vi "18_DC Motor_PID_test_3.vi"() -> ()   [LabVIEW 2018]
uses:
  <userlib>/KNR OS 4.0 LabVIEW Toolkit/Type Definition/DC Motor Port.ctl
  <userlib>/KNR OS 4.0 LabVIEW Toolkit/Type Definition/Resource.ctl
panel:
  in  "R Reverse":bool
  in  "Enable Motor 2":bool
  in  "Enable sync":bool=TRUE
  in  "Kp 3":dbl(slide)=0.2 scale=0.0..0.8
  in  "Ki 3":dbl(slide)=0.05 scale=0.0..0.1
  in  "Kd 3":dbl(slide)=0.02 scale=0.0..0.2
  in  "PID sync":bool=TRUE
  out "Speed (+-100%) 2":dbl
  out "Velocity (cm/sec) 2":dbl
  in  "Port 2":T1=5 items=["DS1"=4, "DS2"=5, "DS3"=6, "DS4"=7]
  out "Velocity (cm/sec) Chart 2":dbl(graph)
  out "Desire Velosity (cm/sec) 2":dbl
  in  "Desire Velosity (cm/sec)":dbl=15.0 format="%#_13g"
  in  "F/B switch":bool=TRUE
  in  "Port":T1=4 items=["DS1"=4, "DS2"=5, "DS3"=6, "DS4"=7]
  out "Velocity (cm/sec) Chart":dbl(graph)
  out "Speed (+-100%)":dbl
  in  "Kd":dbl(slide)=0.02 scale=0.0..0.2
  in  "Ki":dbl(slide)=0.05 scale=0.0..0.1
  in  "Kp":dbl(slide)=0.2 scale=0.0..0.8
  in  "stop":bool
  in  "Enable Motor 1":bool
  out "Velocity (cm/sec)":dbl
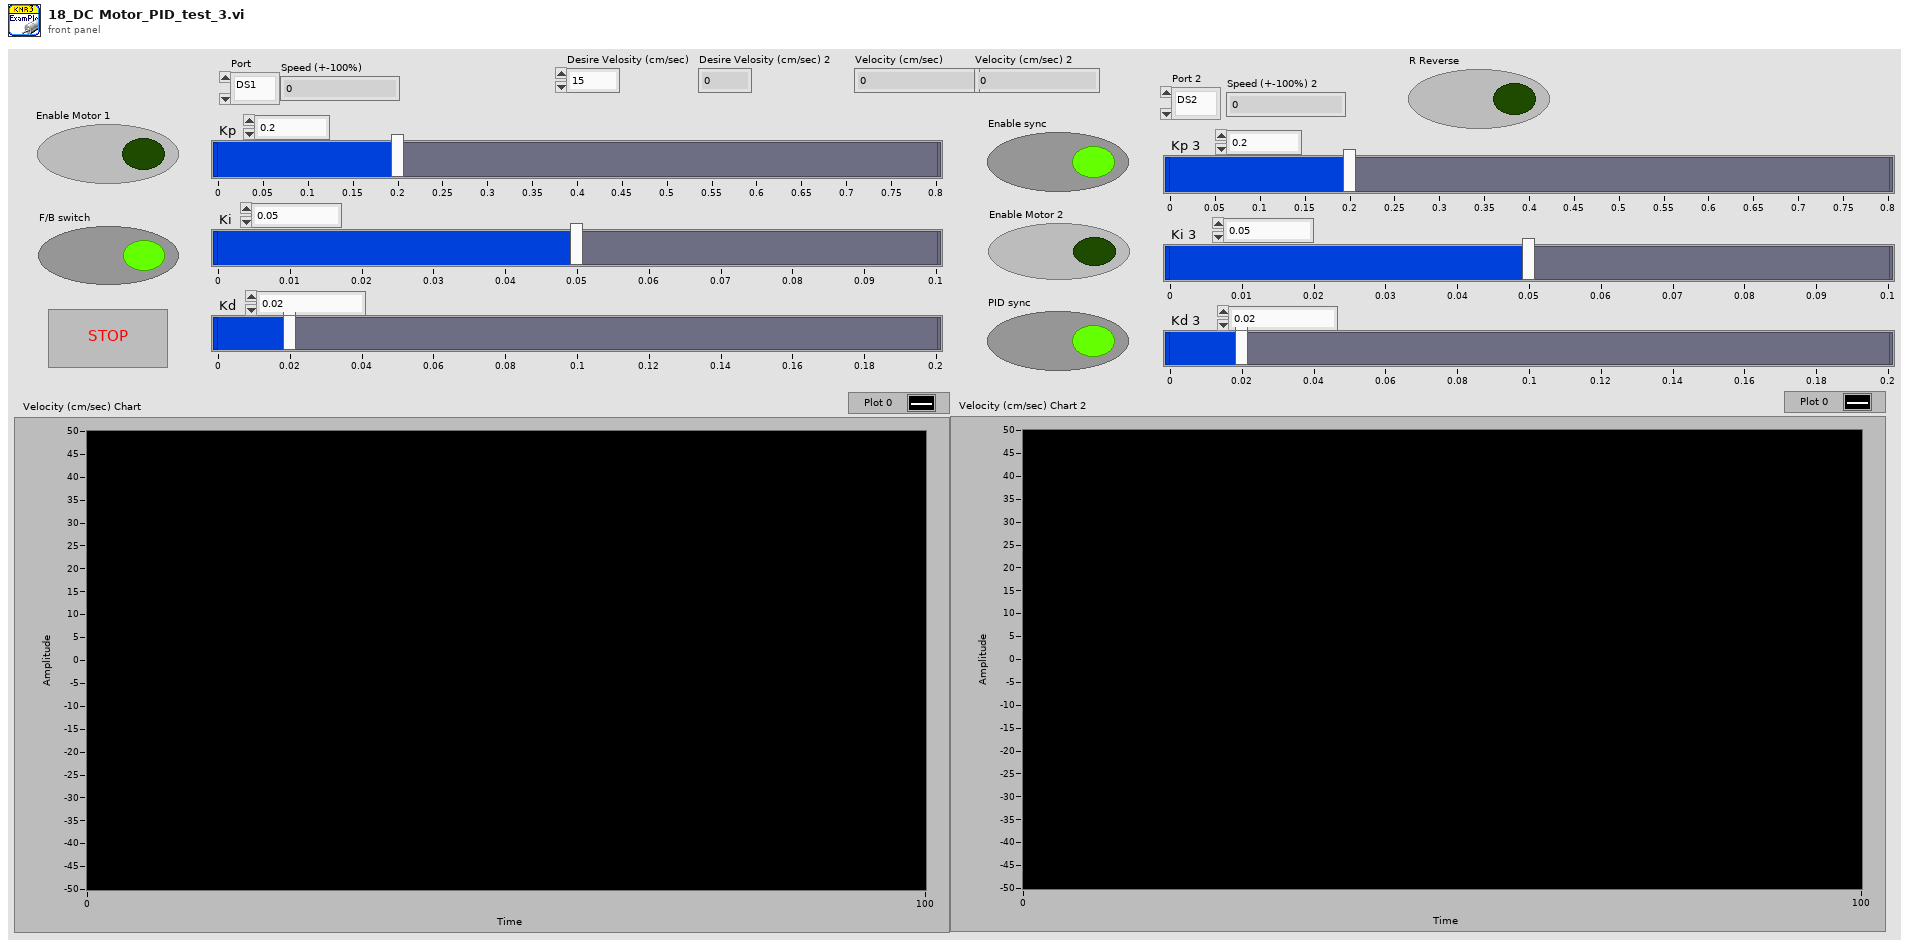
[diagram p1: front panel]
types:
  T1 = typedef "DC Motor Port.ctl" = u16
  T2 = typedef "Resource.ctl" = enum16{"KNRm_DDRC", "KNRm_DDDD", "KNRm_DDDR", "KNRm_DDDC", "KNR", "KNRm_neww"}
  T3 = typedef "KNR3 Reference.ctl" = cluster{"FPGA Session":refnum<class "FPGA Interface Base.lvclass">, "Resource":T2}
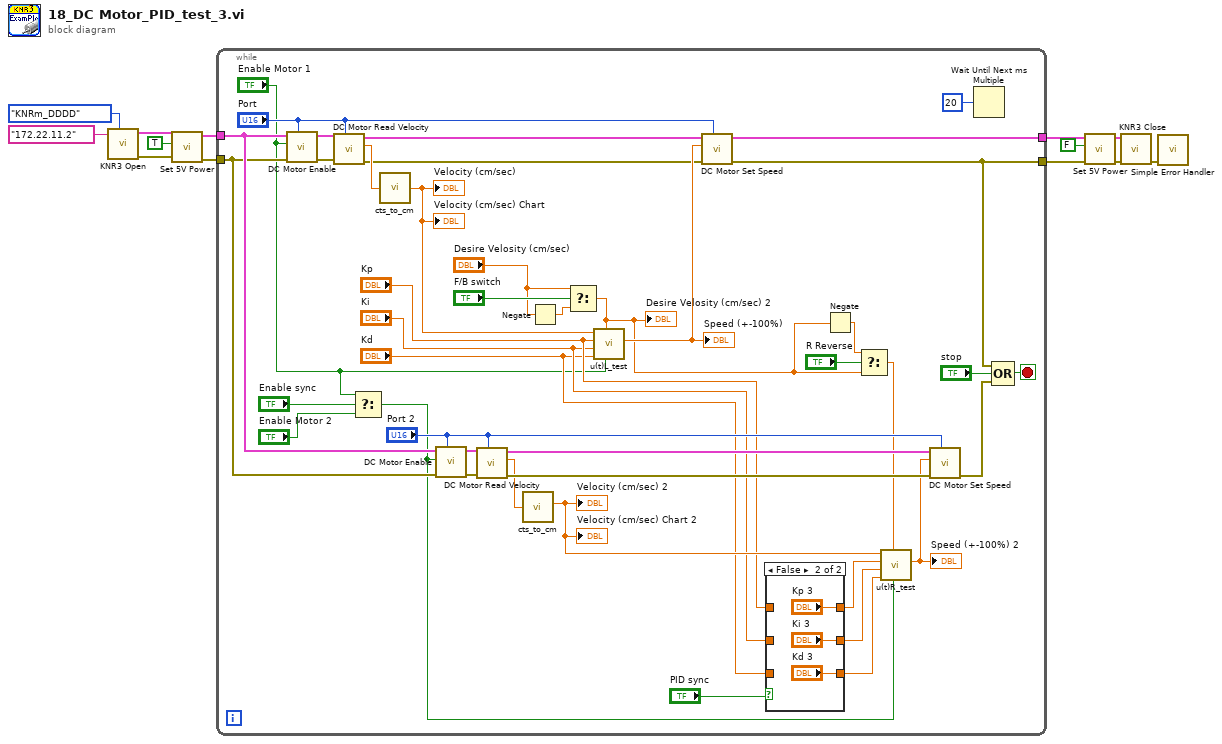
[diagram p0: block diagram]
diagram:
  n1 = call <userlib>:"KNR3 Open.vi"("Resource"=Resource."KNRm_DDDD", "IP"="172.22.11.2") -> ("error out"=w6:errorcluster, "KNR out"=w8:T3)  [unwired: 8 in]
  n2 = call <userlib>:"Set 5V Power.vi"("error in (no error)"=w6, "5V Power(T)"=TRUE ("5V Power"), "KNR in"=w8) -> ("error out"=w10:errorcluster, "KNR out"=w11:T3)  [unwired: 7 in]
  n3 = while {
    tunnel: w11 -> [w36]
    tunnel: w10 -> [w35]
    tunnel: [w47] -> w4
    tunnel: [w46] -> w3
    stop <- w53 stop-if-true
    n4 = call <userlib>:"DC Motor Enable.vi"("Port (DS1)"="Port", "error in (no error)"=w35, "Enable Motor(F)"="Enable Motor 1", "KNR in"=w36) -> ("error out"=w50:errorcluster, "KNR out"=w51:T3)  [unwired: 6 in]
    n5 = call <userlib>:"DC Motor Read Velocity.vi"("Port (DS1)"="Port", "error in (no error)"=w50, "KNR in"=w51) -> ("error out"=w43:errorcluster, "Velocity (cts/sec)"=w49:dbl, "KNR out"=w44:T3)  [unwired: 6 in]
    n6 = Select(t="Enable Motor 1", s="Enable sync", f="Enable Motor 2") -> (s? t:f=w21:bool)
    n7 = call "cts_to_cm.vi"("cts"=w49) -> ("cm"=w28:dbl)
    "Velocity (cm/sec)" <- w28
    "Velocity (cm/sec) Chart" <- w28
    n8 = call <userlib>:"DC Motor Enable.vi"("Port (DS1)"="Port 2", "error in (no error)"=w35, "Enable Motor(F)"=w21, "KNR in"=w36) -> ("error out"=w38:errorcluster, "KNR out"=w37:T3)  [unwired: 6 in]
    n9 = call <userlib>:"DC Motor Read Velocity.vi"("Port (DS1)"="Port 2", "error in (no error)"=w38, "KNR in"=w37) -> ("error out"=w42:errorcluster, "Velocity (cts/sec)"=w39:dbl, "KNR out"=w41:T3)  [unwired: 6 in]
    n10 = call "cts_to_cm.vi"("cts"=w39) -> ("cm"=w31:dbl)
    "Velocity (cm/sec) 2" <- w31
    "Velocity (cm/sec) Chart 2" <- w31
    n11 = Negate(x="Desire Velosity (cm/sec)") -> (-x=w18:dbl)
    n12 = Select(t="Desire Velosity (cm/sec)", s="F/B switch", f=w18) -> (s? t:f=w13:dbl)
    "Desire Velosity (cm/sec) 2" <- w13
    n13 = call "u(t)L_test.vi"("enable"="Enable Motor 1", "Desire Velosity"=w13, "Kd"="Kd", "Ki"="Ki", "Kp"="Kp", "Velocity"=w28) -> ("u(t)"=w45:dbl)  [unwired: 5 in]
    "Speed (+-100%)" <- w45
    n14 = call <userlib>:"DC Motor Set Speed.vi"("Port (DS1)"="Port", "error in (no error)"=w43, "Speed (+-100%)"=w45, "KNR in"=w44) -> ("error out"=w46:errorcluster, "KNR out"=w47:T3)  [unwired: 6 in]
    n15 = case shown="False" "PID sync" {
      tunnel: [w57 "Kp 3"] -> w34
      tunnel: [w55 "Kd 3"] -> w33
      tunnel: [w56 "Ki 3"] -> w32
      tunnel: "Kp" -> [w57 _]
      tunnel: "Ki" -> [w56 _]
      tunnel: "Kd" -> [w55 _]
      frame True {
      }
      frame False {
      }
    }
    n16 = Negate(x=w13) -> (-x=w14:dbl)
    n17 = Select(t=w14, s="R Reverse", f=w13) -> (s? t:f=w16:dbl)
    n18 = call "u(t)R_test.vi"("enable"=w21, "Desire Velosity"=w16, "Kd"=w33, "Ki"=w32, "Kp"=w34, "Velocity"=w31) -> ("u(t)"=w30:dbl)  [unwired: 5 in]
    "Speed (+-100%) 2" <- w30
    n19 = call <userlib>:"DC Motor Set Speed.vi"("Port (DS1)"="Port 2", "error in (no error)"=w42, "Speed (+-100%)"=w30, "KNR in"=w41) -> ("error out"=w17:errorcluster)  [unwired: 6 in, 1 out]
    n20 = Wait Until Next ms Multiple(millisecond multiple=u32 20) -> ()  [unwired: 1 out]
    n21 = Compound Arithmetic op=OR(w46, "stop", w17) -> (w53:bool)
  }
  n22 = call <userlib>:"Set 5V Power.vi"("5V Power(T)"=FALSE, "KNR in"=w4) -> ("KNR out"=w2:T3)  [unwired: 8 in, 1 out]
  n23 = call <userlib>:"KNR3 Close.vi"("error in (no error)"=w3, "KNR in"=w2) -> ("error out"=w9:errorcluster)  [unwired: 9 in]
  n24 = call <vilib>:"Simple Error Handler.vi"("error in (no error)"=w9) -> ()  [unwired: 4 in, 5 out]
